vi "Flatten Variant to JSON Helper.vi"(0 "Variant in":variant, 5 "indent":i32, 7 "enable LabVIEW extensions? (T)":bool=TRUE, 9 "pretty print? (T)":bool=TRUE, 11 "error in (no error)":errorcluster) -> (4 "Variant out":variant, 6 "String":string, 15 "error out":errorcluster)   [LabVIEW 2017, in "Variant JSON API.lvlib"]
uses:
  Variant JSON API.lvlib
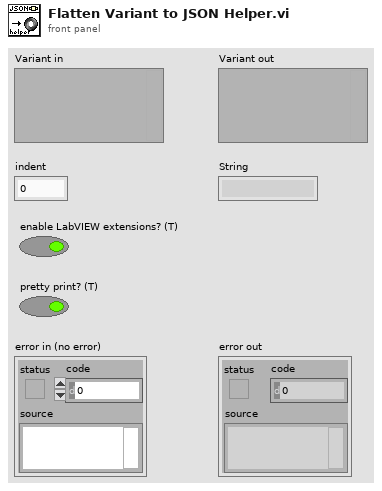
[diagram p1: front panel]
types:
  T1 = typedef "Variant JSON API.lvlib/JSON Type.ctl" = enum16{"String", "Numeric", "Boolean", "NULL", "Object", "Array"}
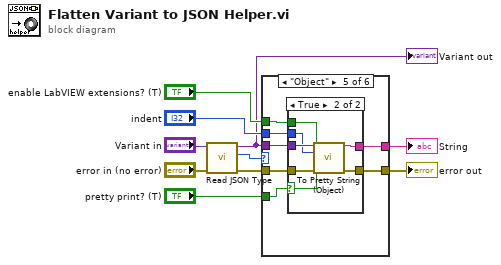
[diagram p0: block diagram]
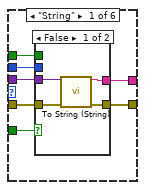
[diagram p2: hidden frame]
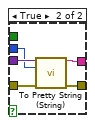
[diagram p3: hidden frame]
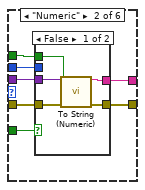
[diagram p4: hidden frame]
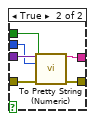
[diagram p5: hidden frame]
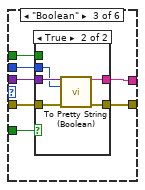
[diagram p6: hidden frame]
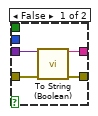
[diagram p7: hidden frame]
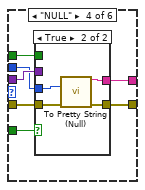
[diagram p8: hidden frame]
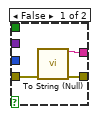
[diagram p9: hidden frame]
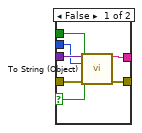
[diagram p10: hidden frame]
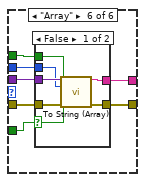
[diagram p11: hidden frame]
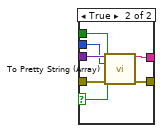
[diagram p12: hidden frame]
diagram:
  n1 = call "Read JSON Type.vi"("error in (no error)"="error in (no error)", "Variant in"="Variant in") -> ("error out"=w2:errorcluster, "datatype"=w1:T1, "JSON Value out"=w4:variant)  [unwired: 7 in]
  "Variant out" <- w4
  n2 = case shown="\"Object\"" w1 {
    tunnel: [w17 w33 w51 w67 w81 w102] -> w10
    tunnel: [w16 w32 w50 w66 w80 w101] -> w9
    tunnel: "enable LabVIEW extensions? (T)" -> [w15 w31 w49 w65 w79 w100]
    tunnel: w2 -> [w14 w30 w48 w64 w78 w99]
    tunnel: w4 -> [w13 w29 w47 w63 w77 w98]
    tunnel: "pretty print? (T)" -> [w12 w27 w46 w62 w76 w97]
    tunnel: "indent" -> [w11 w28 w45 w61 w75 w96]
    frame "String" {
      n3 = case shown="False" w12 {
        tunnel: [w21 w26] -> w17
        tunnel: [w20 w23] -> w16
        tunnel: w15 -> [_ _]
        tunnel: w14 -> [w19 w25]
        tunnel: w13 -> [w18 w24]
        tunnel: w11 -> [_ w22]
        frame False {
          n4 = call "To String (String).vi"("Variant in"=w18, "error in (no error)"=w19) -> ("String"=w20:string, "error out"=w21:errorcluster)  [unwired: 12 in]
        }
        frame True {
          n5 = call "To Pretty String (String).vi"("Variant in"=w24, "indent"=w22, "error in (no error)"=w25) -> ("String"=w23:string, "error out"=w26:errorcluster)  [unwired: 11 in]
        }
      }
    }
    frame "Numeric" {
      n6 = case shown="False" w27 {
        tunnel: [w38 w44] -> w33
        tunnel: [w37 w39] -> w32
        tunnel: w31 -> [w36 w40]
        tunnel: w30 -> [w35 w42]
        tunnel: w29 -> [w34 w43]
        tunnel: w28 -> [_ w41]
        frame False {
          n7 = call "To String (Numeric).vi"("Variant in"=w34, "enable LabVIEW extensions? (T)"=w36, "error in (no error)"=w35) -> ("String"=w37:string, "error out"=w38:errorcluster)  [unwired: 11 in]
        }
        frame True {
          n8 = call "To Pretty String (Numeric).vi"("Variant in"=w43, "indent"=w41, "enable LabVIEW extensions? (T)"=w40, "error in (no error)"=w42) -> ("String"=w39:string, "error out"=w44:errorcluster)  [unwired: 10 in]
        }
      }
    }
    frame "Boolean" {
      n9 = case shown="True" w46 {
        tunnel: [w55 w56] -> w51
        tunnel: [w54 w57] -> w50
        tunnel: w49 -> [_ _]
        tunnel: w48 -> [w53 w60]
        tunnel: w47 -> [w52 w59]
        tunnel: w45 -> [_ w58]
        frame False {
          n10 = call "To String (Boolean).vi"("Variant in"=w52, "error in (no error)"=w53) -> ("String"=w54:string, "error out"=w55:errorcluster)  [unwired: 12 in]
        }
        frame True {
          n11 = call "To Pretty String (Boolean).vi"("Variant in"=w59, "indent"=w58, "error in (no error)"=w60) -> ("String"=w57:string, "error out"=w56:errorcluster)  [unwired: 11 in]
        }
      }
    }
    frame "NULL" {
      n12 = case shown="True" w62 {
        tunnel: [w70 w74] -> w67
        tunnel: [w69 w73] -> w66
        tunnel: w65 -> [_ _]
        tunnel: w64 -> [w68 w72]
        tunnel: w63 -> [_ _]
        tunnel: w61 -> [_ w71]
        frame False {
          n13 = call "To String (Null).vi"("error in (no error)"=w68) -> ("String"=w69:string, "error out"=w70:errorcluster)  [unwired: 13 in]
        }
        frame True {
          n14 = call "To Pretty String (Null).vi"("indent"=w71, "error in (no error)"=w72) -> ("String"=w73:string, "error out"=w74:errorcluster)  [unwired: 12 in]
        }
      }
    }
    frame "Object" {
      n15 = case shown="True" w76 {
        selector: w76 -> [w83 w95]
        tunnel: [w88 w91] -> w81
        tunnel: [w87 w93] -> w80
        tunnel: w79 -> [w86 w92]
        tunnel: w78 -> [w85 w90]
        tunnel: w77 -> [w84 w94]
        tunnel: w75 -> [w82 w89]
        frame False {
          n16 = call "To String (Object).vi"("Variant in"=w84, "indent"=w82, "enable LabVIEW extensions? (T)"=w86, "pretty print? (T)"=w83, "error in (no error)"=w85) -> ("String"=w87:string, "error out"=w88:errorcluster)  [unwired: 9 in]
        }
        frame True {
          n17 = call "To Pretty String (Object).vi"("Variant in"=w94, "indent"=w89, "enable LabVIEW extensions? (T)"=w92, "pretty print? (T)"=w95, "error in (no error)"=w90) -> ("Pretty Print String"=w93:string, "error out"=w91:errorcluster)  [unwired: 9 in]
        }
      }
    }
    frame "Array" {
      n18 = case shown="False" w97 {
        selector: w97 -> [w104 w111]
        tunnel: [w109 w115] -> w102
        tunnel: [w108 w116] -> w101
        tunnel: w100 -> [w107 w112]
        tunnel: w99 -> [w106 w114]
        tunnel: w98 -> [w105 w113]
        tunnel: w96 -> [w103 w110]
        frame False {
          n19 = call "To String (Array).vi"("Variant in"=w105, "indent"=w103, "enable LabVIEW extensions? (T)"=w107, "pretty print? (T)"=w104, "error in (no error)"=w106) -> ("String"=w108:string, "error out"=w109:errorcluster)  [unwired: 9 in]
        }
        frame True {
          n20 = call "To Pretty String (Array).vi"("Variant in"=w113, "indent"=w110, "enable LabVIEW extensions? (T)"=w112, "pretty print? (T)"=w111, "error in (no error)"=w114) -> ("Pretty Print String"=w116:string, "error out"=w115:errorcluster)  [unwired: 9 in]
        }
      }
    }
  }
  "error out" <- w10
  "String" <- w9
